vi "诊断标定3 - 副本.vi"(8 "CAN端口":u16(ring), 9 "设备索引号":u16(ring), 10 "CAN卡类型":u32(ring)=21) -> ()   [LabVIEW 2013] (continued)
      w58 = string[][] [["", "", "", "", "", "", "", "", "", "", "", "", "", "", "", "", "", "", "", "", "", "", "", "", "", "", "", "", "", "", "", "", "", "", "", "", "", "", "", "", ""], ["", "", "", "", "", "", "", "", "", "", "", "", "", "", "", "", "", "", "", "", "", "", "", "", "", "", "", "", "", "", "", "", "", "", "", "", "", "", "", "", ""], ["", "", "", "", "", "", "", "", "", "", "", "", "", "", "", "", "", "", "", "", "", "", "", "", "", "", "", "", "", "", "", "", "", "", "", "", "", "", "", "", ""], ["", "", "", "", "", "", "", "", "", "", "", "", "", "", "", "", "", "", "", "", "", "", "", "", "", "", "", "", "", "", "", "", "", "", "", "", "", "", "", "", ""], ["", "", "", "", "", "", "", "", "", "", "", "", "", "", "", "", "", "", "", "", "", "", "", "", "", "", "", "", "", "", "", "", "", "", "", "", "", "", "", "", ""], ["", "", "", "", "", "", "", "", "", "", "", "", "", "", "", "", "", "", "", "", "", "", "", "", "", "", "", "", "", "", "", "", "", "", "", "", "", "", "", "", ""], ["", "", "", "", "", "", "", "", "", "", "", "", "", "", "", "", "", "", "", "", "", "", "", "", "", "", "", "", "", "", "", "", "", "", "", "", "", "", "", "", ""], ["", "", "", "", "", "", "", "", "", "", "", "", "", "", "", "", "", "", "", "", "", "", "", "", "", "", "", "", "", "", "", "", "", "", "", "", "", "", "", "", ""], ["", "", "", "", "", "", "", "", "", "", "", "", "", "", "", "", "", "", "", "", "", "", "", "", "", "", "", "", "", "", "", "", "", "", "", "", "", "", "", "", ""], ["", "", "", "", "", "", "", "", "", "", "", "", "", "", "", "", "", "", "", "", "", "", "", "", "", "", "", "", "", "", "", "", "", "", "", "", "", "", "", "", ""], ["", "", "", "", "", "", "", "", "", "", "", "", "", "", "", "", "", "", "", "", "", "", "", "", "", "", "", "", "", "", "", "", "", "", "", "", "", "", "", "", ""], ["", "", "", "", "", "", "", "", "", "", "", "", "", "", "", "", "", "", "", "", "", "", "", "", "", "", "", "", "", "", "", "", "", "", "", "", "", "", "", "", ""], ["", "", "", "", "", "", "", "", "", "", "", "", "", "", "", "", "", "", "", "", "", "", "", "", "", "", "", "", "", "", "", "", "", "", "", "", "", "", "", "", ""], ["", "", "", "", "", "", "", "", "", "", "", "", "", "", "", "", "", "", "", "", "", "", "", "", "", "", "", "", "", "", "", "", "", "", "", "", "", "", "", "", ""], ["", "", "", "", "", "", "", "", "", "", "", "", "", "", "", "", "", "", "", "", "", "", "", "", "", "", "", "", "", "", "", "", "", "", "", "", "", "", "", "", ""], ["", "", "", "", "", "", "", "", "", "", "", "", "", "", "", "", "", "", "", "", "", "", "", "", "", "", "", "", "", "", "", "", "", "", "", "", "", "", "", "", ""], ["", "", "", "", "", "", "", "", "", "", "", "", "", "", "", "", "", "", "", "", "", "", "", "", "", "", "", "", "", "", "", "", "", "", "", "", "", "", "", "", ""], ["", "", "", "", "", "", "", "", "", "", "", "", "", "", "", "", "", "", "", "", "", "", "", "", "", "", "", "", "", "", "", "", "", "", "", "", "", "", "", "", ""], ["", "", "", "", "", "", "", "", "", "", "", "", "", "", "", "", "", "", "", "", "", "", "", "", "", "", "", "", "", "", "", "", "", "", "", "", "", "", "", "", ""], ["", "", "", "", "", "", "", "", "", "", "", "", "", "", "", "", "", "", "", "", "", "", "", "", "", "", "", "", "", "", "", "", "", "", "", "", "", "", "", "", ""], ["", "", "", "", "", "", "", "", "", "", "", "", "", "", "", "", "", "", "", "", "", "", "", "", "", "", "", "", "", "", "", "", "", "", "", "", "", "", "", "", ""], ["", "", "", "", "", "", "", "", "", "", "", "", "", "", "", "", "", "", "", "", "", "", "", "", "", "", "", "", "", "", "", "", "", "", "", "", "", "", "", "", ""], ["", "", "", "", "", "", "", "", "", "", "", "", "", "", "", "", "", "", "", "", "", "", "", "", "", "", "", "", "", "", "", "", "", "", "", "", "", "", "", "", ""], ["", "", "", "", "", "", "", "", "", "", "", "", "", "", "", "", "", "", "", "", "", "", "", "", "", "", "", "", "", "", "", "", "", "", "", "", "", "", "", "", ""], ["", "", "", "", "", "", "", "", "", "", "", "", "", "", "", "", "", "", "", "", "", "", "", "", "", "", "", "", "", "", "", "", "", "", "", "", "", "", "", "", ""], ["", "", "", "", "", "", "", "", "", "", "", "", "", "", "", "", "", "", "", "", "", "", "", "", "", "", "", "", "", "", "", "", "", "", "", "", "", "", "", "", ""], ["", "", "", "", "", "", "", "", "", "", "", "", "", "", "", "", "", "", "", "", "", "", "", "", "", "", "", "", "", "", "", "", "", "", "", "", "", "", "", "", ""], ["", "", "", "", "", "", "", "", "", "", "", "", "", "", "", "", "", "", "", "", "", "", "", "", "", "", "", "", "", "", "", "", "", "", "", "", "", "", "", "", ""], ["", "", "", "", "", "", "", "", "", "", "", "", "", "", "", "", "", "", "", "", "", "", "", "", "", "", "", "", "", "", "", "", "", "", "", "", "", "", "", "", ""], ["", "", "", "", "", "", "", "", "", "", "", "", "", "", "", "", "", "", "", "", "", "", "", "", "", "", "", "", "", "", "", "", "", "", "", "", "", "", "", "", ""], ["", "", "", "", "", "", "", "", "", "", "", "", "", "", "", "", "", "", "", "", "", "", "", "", "", "", "", "", "", "", "", "", "", "", "", "", "", "", "", "", ""], ["", "", "", "", "", "", "", "", "", "", "", "", "", "", "", "", "", "", "", "", "", "", "", "", "", "", "", "", "", "", "", "", "", "", "", "", "", "", "", "", ""], ["", "", "", "", "", "", "", "", "", "", "", "", "", "", "", "", "", "", "", "", "", "", "", "", "", "", "", "", "", "", "", "", "", "", "", "", "", "", "", "", ""], ["", "", "", "", "", "", "", "", "", "", "", "", "", "", "", "", "", "", "", "", "", "", "", "", "", "", "", "", "", "", "", "", "", "", "", "", "", "", "", "", ""], ["", "", "", "", "", "", "", "", "", "", "", "", "", "", "", "", "", "", "", "", "", "", "", "", "", "", "", "", "", "", "", "", "", "", "", "", "", "", "", "", ""], ["", "", "", "", "", "", "", "", "", "", "", "", "", "", "", "", "", "", "", "", "", "", "", "", "", "", "", "", "", "", "", "", "", "", "", "", "", "", "", "", ""], ["", "", "", "", "", "", "", "", "", "", "", "", "", "", "", "", "", "", "", "", "", "", "", "", "", "", "", "", "", "", "", "", "", "", "", "", "", "", "", "", ""], ["", "", "", "", "", "", "", "", "", "", "", "", "", "", "", "", "", "", "", "", "", "", "", "", "", "", "", "", "", "", "", "", "", "", "", "", "", "", "", "", ""], ["", "", "", "", "", "", "", "", "", "", "", "", "", "", "", "", "", "", "", "", "", "", "", "", "", "", "", "", "", "", "", "", "", "", "", "", "", "", "", "", ""], ["", "", "", "", "", "", "", "", "", "", "", "", "", "", "", "", "", "", "", "", "", "", "", "", "", "", "", "", "", "", "", "", "", "", "", "", "", "", "", "", ""], ["", "", "", "", "", "", "", "", "", "", "", "", "", "", "", "", "", "", "", "", "", "", "", "", "", "", "", "", "", "", "", "", "", "", "", "", "", "", "", "", ""]]
      w47 = TRUE
      w42 = u32 16777215
      w38 = FALSE ("判定2")
      n3 = control-ref of="结果"() -> (w43:refnum<vi>)
      n4 = control-ref of="模块软件版本 2"() -> (w44:refnum<vi>)
      n5 = control-ref of="结果"() -> (w45:refnum<vi>)
      n6 = control-ref of="单选选项2"() -> (w62:refnum<vi>)
      n7 = control-ref of="单选选项1"() -> (w63:refnum<vi>)
      n8 = local write "key names"(string[] []) -> ()
      n9 = property on="项目信息" class="Tbl (严格)"("Disabled"=w39) -> ()  [unwired: 2 in, 2 out]
      n10 = property on="电池实际容量(A)" class="DigNum (严格)"("Disabled"=w39) -> ()  [unwired: 2 in, 2 out]
      n11 = property on="使用者" class="DigNum (严格)"("Disabled"=w39) -> ()  [unwired: 2 in, 2 out]
      n12 = property on="SOH(%)" class="DigNum (严格)"("Disabled"=w39) -> ()  [unwired: 2 in, 2 out]
      n13 = property on="电池额定容量(A)" class="DigNum (严格)"("Disabled"=w39) -> ()  [unwired: 2 in, 2 out]
      n14 = local write "主从选择"(enum32{"主板", "从板"}."主板" ("主从选择")) -> ()
      n15 = property on="SOC(%)" class="DigNum (严格)"("Disabled"=w39) -> ()  [unwired: 2 in, 2 out]
      n16 = local write "等级 2"(T19."从板信息" ("等级 2")) -> ()
      n17 = local write "主板2"(T8."项目信息" ("主从板")) -> ()
      n18 = property class="MCListbox (严格)"(reference=w45, "ItemNames"=w40) -> ()  [unwired: 1 in, 2 out]
      n19 = property class="MCListbox (严格)"(reference=w44, "ItemNames"=w40) -> ()  [unwired: 1 in, 2 out]
      n20 = property class="MCListbox (严格)"(reference=w43, "ItemNames"=w40) -> ()  [unwired: 1 in, 2 out]
      n21 = property class="Bool (严格)"(reference=w62, "BoolText.TextColor"=u32 87470) -> ()  [unwired: 1 in, 2 out]
      n22 = property class="Bool (严格)"(reference=w63, "BoolText.TextColor"=w42) -> ()  [unwired: 1 in, 2 out]
      n23 = property on="从板号" class="DigNum (严格)"("NumText.BGColor"=w42) -> ()  [unwired: 2 in, 2 out]
      n24 = local write "主从板"(enum32{"单选选项2", "单选选项1"}."单选选项1" ("主从板")) -> ()
      n25 = property on="项目信息2" class="Clust (严格)"("DisabledEnum"=w39) -> ()  [unwired: 2 in, 2 out]
      n26 = property on="系统时钟" class="Str"("Disabled"=w39) -> ()  [unwired: 2 in, 2 out]
      n27 = property on="配置文件版本" class="Str"("Disabled"=w39) -> ()  [unwired: 2 in, 2 out]
      n28 = property on="车架(牌)号" class="Str"("Disabled"=w39) -> ()  [unwired: 2 in, 2 out]
      n29 = property on="产品编号" class="Str"("Disabled"=w39) -> ()  [unwired: 2 in, 2 out]
      n30 = local write "判定3"(w47) -> ()
      n31 = local write "清BUFF"(w47) -> ()
      n32 = local write "1"(w47) -> ()
      n33 = property on="从板个数" class="DigNum (严格)"("Visible"=w47) -> ()  [unwired: 2 in, 2 out]
      n34 = property on="从板个数" class="DigNum (严格)"("NumText.BGColor"=u32 16448250) -> ()  [unwired: 2 in, 2 out]
      n35 = Not(x=w47) -> (.not. x?=w66:bool)
      n36 = local write "布尔"(w47) -> ()
      n37 = property on="主板选项" class="Tree (严格)"("Visible"=w47) -> ()  [unwired: 2 in, 2 out]
      n38 = property on="全部写入" class="Bool (严格)"("DisabledEnum"=2) -> ()  [unwired: 2 in, 2 out]
      n39 = property on="从板选项" class="Tree (严格)"("Visible"=w66) -> ()  [unwired: 2 in, 2 out]
      n40 = property on="当前从板板号" class="DigNum (严格)"("Visible"=w66) -> ()  [unwired: 2 in, 2 out]
      n41 = control-ref of="结果"() -> (w53:refnum<vi>)
      n42 = control-ref of="结果"() -> (w50:refnum<vi>)
      n43 = local write "强制停止版本读取"(w38) -> ()
      n44 = local write "强制终止读写标记"(w38) -> ()
      n45 = control-ref of="项目信息"() -> (w51:refnum<vi>)
      n46 = local write "判定2"(w38) -> ()
      n47 = local write "停止"(w38) -> ()
      n48 = local write "控制1"(w38) -> ()
      n49 = local write "消除"(w38) -> ()
      n50 = global write "EV05全局变量1.vi" "授权功能"(w38) -> ()
      n51 = local write "继电器超时处理"(w38) -> ()
      n52 = local write "1 6"(w38) -> ()
      n53 = local write "1 7"(w38) -> ()
      n54 = local write "1 8"(w38) -> ()
      n55 = local write "1 9"(w38) -> ()
      n56 = local write "1 10"(w38) -> ()
      n57 = local write "1 2"(w38) -> ()
      n58 = local write "1 3"(w38) -> ()
      n59 = local write "1 4"(w38) -> ()
      n60 = local write "1 5"(w38) -> ()
      n61 = local write "1 11"(w38) -> ()
      n62 = for {
        N: 150 -> [_]
        tunnel: w53 -> [w92]
        i -> [w90]
        n63 = Bundle(w90, 0) -> (w88:cluster{i32, i32})  [unwired: 1 out]
        n64 = property class="MCListbox (严格)"(reference=w92, "ActiveCell"=w88, "CellBG"=u32 16448250) -> ()  [unwired: 1 in, 2 out]
      }
      n65 = for {
        N: 150 -> [_]
        tunnel: w51 -> [w87]
        i -> [w86]
        n66 = Bundle(w86, 0) -> (w84:cluster{i32, i32})  [unwired: 1 out]
        n67 = property class="Tbl (严格)"(reference=w87, "Active Cell"=w84, "Cell BG Color"=u32 16448250) -> ()  [unwired: 1 in, 2 out]
      }
      n68 = for {
        N: 150 -> [_]
        tunnel: w50 -> [w97]
        i -> [w95]
        n69 = Bundle(w95, 0) -> (w93:cluster{i32, i32})  [unwired: 1 out]
        n70 = property class="MCListbox (严格)"(reference=w97, "ActiveCell"=w93, "CellBG"=u32 16448250) -> ()  [unwired: 1 in, 2 out]
      }
      n71 = stacked-sequence {
        tunnel: [_ w71] -> w46
        frame #0 {
          n72 = local read "设备索引号"() -> (w68:u16)
          n73 = local read "CAN卡类型"() -> (w67:u32)
          n74 = local read "CAN端口"() -> (w69:u16)
          n75 = dll-call lib="PTH1|abs FBluewave New EnergySVN_WorkBMS_Monitor_Bnet01trunkBMS_Monitor_增加二维码data\nkerneldlls\nusbcan.dll" fn="VCI_ClearBuffer"("DeviceType"=w67, "DeviceInd"=w68, "CANInd"=w69) -> (error out=w70:errorcluster)  [unwired: 4 in, 4 out]
          n76 = call <vilib>:"Clear Errors.vi"("error in (no error)"=w70) -> ()  [unwired: 6 in, 1 out]
        }
        frame #1 {
          w78 = u8 0 items=["Normal", "Listen Only"] ("工作方式")
          w77 = u8 1 items=["Dual Filter", "Single Filter"] ("滤波方式")
          n77 = local read "设备索引号"() -> (w73:u16)
          n78 = local read "CAN卡类型"() -> (w72:u32)
          n79 = local read "CAN端口"() -> (w74:u16)
          n80 = call "CAN_Init-8.6.vi"("CAN卡类型"=w72, "设备索引号"=w73, "CAN端口"=w74, "操作类型"=enum16{"初始化CAN", "关闭CAN"}."初始化CAN", "滤波方式"=w77, "Accept Code"=u32 3221225472, "簇"=T21 {"打开CAN"=FALSE, "初始化CAN"=TRUE, "开始CAN"=TRUE, "重启"=FALSE, "关闭CAN"=FALSE}, "Mask Code"=u32 1073741823 ("Accept Code"), "工作方式"=w78, "是否滤波"=TRUE, "滤波选择"=T20 {"fiter_mode"=1, "fiter_endid"=402653184, "fiter_startid"=419430399}) -> ("error out"=w71:errorcluster)  [unwired: 3 in, 5 out]
        }
      }
      n81 = local write "加热继电器(从)"(w38) -> ()
      n82 = local write "风机继电器(从)"(w38) -> ()
      n83 = local write "DO1"(w38) -> ()
      n84 = local write "DO2"(w38) -> ()
      n85 = local write "DO1 2"(w38) -> ()
      n86 = local write "正级继电器"(w38) -> ()
      n87 = local write "负级继电器"(w38) -> ()
      n88 = local write "加热继电器"(w38) -> ()
      n89 = local write "充电继电器"(w38) -> ()
      n90 = local write "风机继电器"(w38) -> ()
      n91 = local write "预充电继电器"(w38) -> ()
      n92 = property on="保存版本信息" class="Bool (严格)"("Visible"=w38) -> ()  [unwired: 2 in, 2 out]
      n93 = property on="单个读取" class="Bool (严格)"("Visible"=w38) -> ()  [unwired: 2 in, 2 out]
      n94 = property on="单个写入" class="Bool (严格)"("Visible"=w38) -> ()  [unwired: 2 in, 2 out]
      n95 = local write "正级继电器 12"(w38) -> ()
      n96 = local write "正级继电器 2"(w38) -> ()
      n97 = local write "正级继电器 3"(w38) -> ()
      n98 = local write "正级继电器 4"(w38) -> ()
      n99 = local write "正级继电器 5"(w38) -> ()
      n100 = local write "正级继电器 6"(w38) -> ()
      n101 = local write "正级继电器 7"(w38) -> ()
      n102 = local write "正级继电器 8"(w38) -> ()
      n103 = local write "正级继电器 9"(w38) -> ()
      n104 = local write "正级继电器 10"(w38) -> ()
      n105 = local write "正级继电器 11"(w38) -> ()
      n106 = property on="从板号" class="DigNum (严格)"("Visible"=w38) -> ()  [unwired: 2 in, 2 out]
      "电池故障" <- w40
      "模块版本值" <- w58
      "硬件版本" <- w59
      "模块版本名称" <- w58
      "平台软件版本" <- w59
      "项目软件版本" <- w59
      "模块个数" <- u8[] [0, 0, 0, 0, 0, 0, 0, 0, 0, 0, 0, 0, 0, 0, 0, 0, 0, 0, 0, 0, 0, 0, 0, 0, 0, 0, 0, 0, 0, 0, 0, 0] ("模块个数")
    }
  }
  n107 = stacked-sequence {
    tunnel: [w98] -> w23
    frame #0 {
      n108 = call <vilib>:"Set Busy.vi"() -> ()  [unwired: 10 in, 2 out]
      n109 = disable-structure shown="禁用" {
        frame Disabled {
          n110 = control-ref of="主板选项"() -> (w217:refnum<vi>)
          n111 = stacked-sequence {
            tunnel: w217 -> [w219 w377 w415]
            frame #0 {
              # "加热和充电控制参数"
              n112 = global read "功能码全局.vi" "主板控制类信息10"() -> (w229:bool[])
              n113 = Index Array(array=w229) -> (element #5=w223:bool, element #6=w221:bool, element #7=w222:bool, element #8=w220:bool)  [unwired: 8 in, 4 out]
              n114 = Not Or(1:w222, 2:w223) -> (0:w228:bool)
              n115 = Not Or(1:w220, 2:w221) -> (0:w226:bool)
              n116 = for {
                N: 8 -> [_]
                tunnel: w219 -> [w349]
                tunnel: w228 -> [w345]
                tunnel: [w344] -> w227
                i -> [w347]
                n117 = Add(x=w347, y=69) -> (x+y=w348:i32)
                n118 = property class="Tree (严格)"(reference=w349, "Active Item Row Number"=w348, "Disabled?"=w345) -> (error out=w344:errorcluster)  [unwired: 1 in, 1 out]
              }
              n119 = for {
                N: 9 -> [_]
                tunnel: w219 -> [w343]
                tunnel: w226 -> [w339]
                tunnel: w227 -> [w338]
                tunnel: [w337] -> w218
                i -> [w341]
                n120 = Add(x=w341, y=77) -> (x+y=w342:i32)
                n121 = property class="Tree (严格)"(reference=w343, error in=w338, "Active Item Row Number"=w342, "Disabled?"=w339) -> (error out=w337:errorcluster)  [unwired: 1 out]
              }
              n122 = stacked-sequence {
                tunnel: w219 -> [w249 _ _]
                tunnel: w218 -> [w248 _ _]
                frame #0 {
                  # "电池信息"
                  n123 = global read "功能码全局.vi" "主板版本号11"() -> (w250:bool[])
                  n124 = global read "功能码全局.vi" "主板项目信息4"() -> (w232:bool[])
                  n125 = Index Array(array=w250) -> (element #1=w246:bool, element #2=w245:bool, element #3=w239:bool, element #4=w233:bool, element #6=w238:bool, element #7=w237:bool, element #8=w236:bool)  [unwired: 8 in, 1 out]
                  n126 = Index Array(array=w232, index=4 ("索引")) -> (element=w230:bool)
                  n127 = Or(x=w239, y=w233) -> (x .or. y?=w234:bool)
                  n128 = Not(x=w237) -> (.not. x?=w241:bool)
                  n129 = Not(x=w236) -> (.not. x?=w240:bool)
                  n130 = Not(x=w238) -> (.not. x?=w242:bool)
                  n131 = property on="硬件版本号" class="Str"("Visible"=w239) -> ()  [unwired: 2 in, 2 out]
                  n132 = property on="读硬件版本号" class="Bool (严格)"("Visible"=w239) -> ()  [unwired: 2 in, 2 out]
                  n133 = property on="项目软件版本号" class="Str"("Visible"=w239) -> ()  [unwired: 2 in, 2 out]
                  n134 = property on="项目软本读取" class="Bool (严格)"("Visible"=w239) -> ()  [unwired: 2 in, 2 out]
                  n135 = property on="继电器屏1 2" class="TabCtl (严格)"("Visible"=w242) -> ()  [unwired: 2 in, 2 out]
                  n136 = property on="均衡屏" class="TabCtl (严格)"("Visible"=w240) -> ()  [unwired: 2 in, 2 out]
                  n137 = property on="继电器屏1 2" class="TabCtl (严格)"("Visible"=w242) -> ()  [unwired: 2 in, 2 out]
                  n138 = property on="DO屏" class="TabCtl (严格)"("Visible"=w241) -> ()  [unwired: 2 in, 2 out]
                  n139 = Compound Arithmetic op=OR(w238, w237, w236) -> (w235:bool)
                  n140 = Not Or(1:w245, 2:w246) -> (0:w244:bool)
                  n141 = stacked-sequence {
                    tunnel: w235 -> [_ w255 _]
                    tunnel: w234 -> [_ _ w259]
                    tunnel: w230 -> [w251 _ _]
                    frame #0 {
                      n142 = case shown="真" w251 {
                        frame False {
                        }
                        frame True {
                          n143 = local write "主界面选项"(enum32{"单选选项1", "单选选项2", "单选选项2 2", "单选选项2 3"}."单选选项2 3" ("主界面选项")) -> ()
                          n144 = local write "面板选择"(T7."高压板校正" ("面板选择")) -> ()
                        }
                      }
                      n145 = control-ref of="单选选项2 3"() -> (w252:refnum<vi>)
                      n146 = property class="Bool (严格)"(reference=w252, "Visible"=w251) -> ()  [unwired: 1 in, 2 out]
                    }
                    frame #1 {
                      n147 = control-ref of="单选选项2 2"() -> (w256:refnum<vi>)
                      n148 = case shown="真" w255 {
                        frame False {
                        }
                        frame True {
                          n149 = local write "主界面选项"(enum32{"单选选项1", "单选选项2", "单选选项2 2", "单选选项2 3"}."单选选项2 2" ("主界面选项")) -> ()
                          n150 = local write "面板选择"(enum32{"读写参数", "版本读取", "其它诊断"}."其它诊断" ("选项卡控件 2")) -> ()
                        }
                      }
                      n151 = property class="Bool (严格)"(reference=w256, "Visible"=w255) -> ()  [unwired: 1 in, 2 out]
                    }
                    frame #2 {
                      n152 = control-ref of="单选选项2"() -> (w260:refnum<vi>)
                      n153 = case shown="真" w259 {
                        frame False {
                        }
                        frame True {
                          n154 = local write "主界面选项"(enum32{"单选选项1", "单选选项2", "单选选项2 2", "单选选项2 3"}."单选选项2" ("主界面选项")) -> ()
                          n155 = local write "面板选择"(enum32{"读写参数", "版本读取", "其它诊断"}."版本读取" ("选项卡控件 2")) -> ()
                        }
                      }
                      n156 = property class="Bool (严格)"(reference=w260, "Visible"=w259) -> ()  [unwired: 1 in, 2 out]
                    }
                  }
                  n157 = for {
                    N: 5 -> [_]
                    tunnel: w249 -> [w269]
                    tunnel: w244 -> [w265]
                    tunnel: w248 -> [w264]
                    tunnel: [w263] -> w247
                    i -> [w267]
                    n158 = Add(x=w267, y=86) -> (x+y=w268:i32)
                    n159 = property class="Tree (严格)"(reference=w269, error in=w264, "Active Item Row Number"=w268, "Disabled?"=w265) -> (error out=w263:errorcluster)  [unwired: 1 out]
                  }
                  n160 = property on="模块软件版本 2" class="MCListbox (严格)"("Visible"=w233) -> ()  [unwired: 2 in, 2 out]
                  n161 = property on="模块软件版本" class="Enum (严格)"("Visible"=w233) -> ()  [unwired: 2 in, 2 out]
                  n162 = property on="平台软件版本号" class="Str"("Visible"=w233) -> ()  [unwired: 2 in, 2 out]
                  n163 = property on="模块版本读取" class="Bool (严格)"("Visible"=w233) -> ()  [unwired: 2 in, 2 out]
                  n164 = property on="平台软件版本读取" class="Bool (严格)"("Visible"=w233) -> ()  [unwired: 2 in, 2 out]
                  n165 = call <vilib>:"Clear Errors.vi"("error in (no error)"=w247) -> ()  [unwired: 6 in, 1 out]
                }
                frame #1 {
                  n166 = global read "功能码全局.vi" "主板项目信息7"() -> (w309:bool[])
                  n167 = global read "功能码全局.vi" "主板控制类信息10"() -> (w305:bool[])
                  n168 = global read "功能码全局.vi" "主板故障阀值9"() -> (w308:bool[])
                  n169 = global read "功能码全局.vi" "主板项目信息4"() -> (w287:bool[])
                  n170 = global read "功能码全局.vi" "主板项目信息5"() -> (w296:bool[])
                  n171 = global read "功能码全局.vi" "主板项目信息6"() -> (w286:bool[])
                  n172 = global read "功能码全局.vi" "主板版本号11"() -> (w295:bool[])
                  n173 = Delete From Array(array=w286, length=1 ("长度"), index=0 ("索引")) -> (deleted portion=w297:bool[], array with subset deleted=w313:bool[])
                  n174 = Index Array(array=w287, index #1=5 ("索引"), index #2=6 ("索引"), index #3=7 ("索引")) -> (element #1=w298:bool, element #2=w314:bool, element #3=w270:bool)
                  n175 = Index Array(array=w295) -> (element #1=w302:bool, element #2=w318:bool)  [unwired: 2 in]
                  n176 = Array Subset(array=w308, index=2 ("索引"), length=3 ("长度")) -> (w300:bool[])
                  n177 = Delete From Array(array=w309, length=3 ("索引"), index=2 ("长度")) -> (deleted portion=w299:bool[], array with subset deleted=w315:bool[])
                  n178 = Array Subset(array=w305, index=4 ("索引"), length=2 ("长度")) -> (w301:bool[])
                  n179 = global read "功能码全局.vi" "18"() -> (w278:bool[])
                  n180 = global read "功能码全局.vi" "16"() -> (w279:bool[])
                  n181 = Insert Into Array(array=w296, new element #1=w297, new element #2=w298, new element #3=w299, new element #4=w300, new element #5=w301, new element #6=w302) -> (w319:bool[])  [unwired: 1 in]
                  n182 = Array Subset(array=w305, index=6 ("索引"), length=2 ("长度")) -> (w317:bool[])
                  n183 = Array Subset(array=w308, index=5 ("索引"), length=3 ("长度")) -> (w316:bool[])
                  n184 = And Array Elements(Boolean array=w319) -> (logical AND=w284:bool)
                  n185 = Array Subset(array=w278, index=0 ("索引"), length=8 ("长度")) -> (w276:bool[])
                  n186 = Array Subset(array=w279, index=4 ("索引"), length=4 ("长度")) -> (w275:bool[])
                  n187 = Or Array Elements(Boolean array=w319) -> (logical OR=w271:bool)
                  n188 = Insert Into Array(array=w313, new element #1=w314, new element #2=w315, new element #3=w316, new element #4=w317, new element #5=w318) -> (w320:bool[])  [unwired: 1 in]
                  n189 = property on="全部读取" class="Bool (严格)"("Visible"=w284) -> ()  [unwired: 2 in, 2 out]
                  n190 = global read "功能码全局.vi" "15"() -> (w277:bool[])
                  n191 = And Array Elements(Boolean array=w320) -> (logical AND=w285:bool)
                  n192 = property on="全部写入" class="Bool (严格)"("Visible"=w285) -> ()  [unwired: 2 in, 2 out]
                  n193 = Or Array Elements(Boolean array=w320) -> (logical OR=w321:bool)
                  n194 = Insert Into Array(array=w277, new element #1=w276, new element #2=w275) -> (w274:bool[])  [unwired: 1 in]
                  n195 = Or Array Elements(Boolean array=w274) -> (logical OR=w273:bool)
                  n196 = Compound Arithmetic op=OR(w270, w271, w321, w273) -> (w322:bool)
                  n197 = case shown="真" w322 {
                    frame False {
                    }
                    frame True {
                      n198 = local write "主界面选项"(enum32{"单选选项1", "单选选项2", "单选选项2 2", "单选选项2 3"}."单选选项1" ("主界面选项")) -> ()
                      n199 = local write "面板选择"(enum32{"读写参数", "版本读取", "其它诊断"}."读写参数" ("选项卡控件 2")) -> ()
                    }
                  }
                  n200 = property on="单选选项1" class="Bool (严格)"("Visible"=w322) -> ()  [unwired: 2 in, 2 out]
                }
                frame #2 {
                  n201 = control-ref of="单选选项2 2"() -> (w329:refnum<vi>)
                  n202 = control-ref of="单选选项2 3"() -> (w325:refnum<vi>)
                  n203 = control-ref of="单选选项2"() -> (w331:refnum<vi>)
                  n204 = control-ref of="单选选项1"() -> (w330:refnum<vi>)
                  n205 = local read "主界面选项"() -> (w334:enum32{"单选选项1", "单选选项2", "单选选项2 2", "单选选项2 3"})
                  n206 = Build Array(w330, w331, w329, w325) -> (w328:refnum<vi>[])
                  n207 = Delete From Array(array=w328, index=w334) -> (deleted portion=w332:refnum<vi>, array with subset deleted=w333:refnum<vi>[])  [unwired: 1 in]
                  n208 = property class="Bool (严格)"(reference=w332, "BoolText.TextColor"=u32 87470) -> ()  [unwired: 1 in, 2 out]
                  n209 = for {
                    tunnel: u32 16777215 -> [w336]
                    tunnel: w333 -> [w335] mode=indexing
                    n210 = property class="Bool (严格)"(reference=w335, "BoolText.TextColor"=w336) -> ()  [unwired: 1 in, 2 out]
                  }
                }
              }
            }
            frame #1 {
              # "项目信息"
              # "SOC"
              # "SOH"
              # "电池额定实际容量"
              # "车牌号"
              # "产品编号"
              # "电压个数"
              # "通道电压数"
              # "温度个数"
              # "电压起始值"
              # "温度起始值"
              # "配置文件版本"
              # "系统时钟"
              # "校正时钟"
              n211 = global read "功能码全局.vi" "主板项目信息5"() -> (w410:bool[])
              n212 = global read "功能码全局.vi" "主板项目信息6"() -> (w409:bool[])
              n213 = global read "功能码全局.vi" "主板项目信息7"() -> (w386:bool[])
              n214 = global read "功能码全局.vi" "主板项目信息4"() -> (w357:bool[])
              n215 = Index Array(array=w410) -> (element #1=w407:bool, element #2=w404:bool, element #3=w401:bool, element #4=w398:bool, element #5=w394:bool, element #6=w392:bool, element #7=w389:bool, element #8=w385:bool)  [unwired: 8 in]
              n216 = Index Array(array=w409) -> (element #1=w382:bool, element #2=w406:bool, element #3=w403:bool, element #4=w400:bool, element #5=w397:bool, element #6=w393:bool, element #7=w391:bool, element #8=w388:bool)  [unwired: 8 in]
              n217 = Index Array(array=w386) -> (element #1=w384:bool, element #2=w381:bool, element #3=w379:bool, element #4=w374:bool, element #5=w371:bool, element #6=w378:bool, element #7=w372:bool, element #8=w370:bool)  [unwired: 8 in]
              n218 = Index Array(array=w357) -> (element #6=w353:bool, element #7=w352:bool, element #8=w356:bool)  [unwired: 8 in, 5 out]
              n219 = Not(x=w356) -> (.not. x?=w355:bool)
              n220 = Not Or(1:w352, 2:w353) -> (0:w351:bool)
              n221 = Not Or(1:w406, 2:w407) -> (0:w369:bool)
              n222 = Not Or(1:w403, 2:w404) -> (0:w368:bool)
              n223 = Not Or(1:w400, 2:w401) -> (0:w367:bool)
              n224 = Not Or(1:w397, 2:w398) -> (0:w366:bool)
              n225 = Not Or(1:w393, 2:w394) -> (0:w365:bool)
              n226 = Not Or(1:w391, 2:w392) -> (0:w364:bool)
              n227 = Not Or(1:w388, 2:w389) -> (0:w363:bool)
              n228 = Not Or(1:w384, 2:w385) -> (0:w362:bool)
              n229 = Not Or(1:w378, 2:w379) -> (0:w360:bool)
              n230 = Not Or(1:w370, 2:w371) -> (0:w358:bool)
              n231 = Not Or(1:w372, 2:w374) -> (0:w359:bool)
              n232 = Not Or(1:w381, 2:w382) -> (0:w361:bool)
              n233 = Compound Arithmetic op=OR(w355, w369, w368, w367, w366, w365, w364, w363, w362, w361, w360, w359, w358) -> (w350:bool)
              "项目信息结果" <- w350
              n234 = property class="Tree (严格)"(reference=w377, "Active Item Row Number"=9 ("活动项:行数"), "Disabled?"=w351, "Active Item Row Number"=1 ("活动项:行数"), "Disabled?"=w350, "Active Item Row Number"=0 ("活动项:行数"), "Disabled?"=w355, "Active Item Row Number"=3 ("活动项:行数"), "Disabled?"=w369, "Active Item Row Number"=4 ("活动项:行数"), "Disabled?"=w368, "Active Item Row Number"=5 ("活动项:行数"), "Disabled?"=w367, "Active Item Row Number"=6 ("活动项:行数"), "Disabled?"=w366, "Active Item Row Number"=7 ("活动项:行数"), "Disabled?"=w365, "Active Item Row Number"=8 ("活动项:行数"), "Disabled?"=w364, "Active Item Row Number"=11 ("活动项:行数"), "Disabled?"=w363, "Active Item Row Number"=12 ("活动项:行数"), "Disabled?"=w362, "Active Item Row Number"=13 ("活动项:行数"), "Disabled?"=w361, "Active Item Row Number"=2 ("活动项:行数"), "Disabled?"=w360, "Active Item Row Number"=10 ("活动项:行数"), "Disabled?"=w359, "Active Item Row Number"=14 ("活动项:行数"), "Disabled?"=w358) -> ()  [unwired: 1 in, 2 out]
            }
            frame #2 {
              w420 = 18
              # "一二三级故障"
              n235 = global read "功能码全局.vi" "主板故障阀值9"() -> (w426:bool[])
              n236 = Index Array(array=w426) -> (element #3=w425:bool, element #4=w422:bool, element #5=w419:bool, element #6=w424:bool, element #7=w421:bool, element #8=w418:bool)  [unwired: 8 in, 2 out]
              n237 = Not Or(1:w424, 2:w425) -> (0:w414:bool)
              n238 = Not Or(1:w421, 2:w422) -> (0:w412:bool)
              n239 = Not Or(1:w418, 2:w419) -> (0:w413:bool)
              n240 = for {
                N: w420 -> [_]
                tunnel: w415 -> [w446]
                tunnel: w414 -> [w442]
                tunnel: [w441] -> w423
                i -> [w444]
                n241 = Add(x=w444, y=15) -> (x+y=w445:i32)
                n242 = property class="Tree (严格)"(reference=w446, "Active Item Row Number"=w445, "Disabled?"=w442) -> (error out=w441:errorcluster)  [unwired: 1 in, 1 out]
              }
              n243 = for {
                N: w420 -> [_]
                tunnel: w415 -> [w440]
                tunnel: w412 -> [w436]
                tunnel: w423 -> [w435]
                tunnel: [w434] -> w417
                i -> [w438]
                n244 = Add(x=w438, y=33) -> (x+y=w439:i32)
                n245 = property class="Tree (严格)"(reference=w440, error in=w435, "Active Item Row Number"=w439, "Disabled?"=w436) -> (error out=w434:errorcluster)  [unwired: 1 out]
              }
              n246 = for {
                N: w420 -> [_]
                tunnel: w415 -> [w433]
                tunnel: w413 -> [w429]
                tunnel: w417 -> [w428]
                tunnel: [w427] -> w416
                i -> [w431]
                n247 = Add(x=w431, y=51) -> (x+y=w432:i32)
                n248 = property class="Tree (严格)"(reference=w433, error in=w428, "Active Item Row Number"=w432, "Disabled?"=w429) -> (error out=w427:errorcluster)  [unwired: 1 out]
              }
              n249 = call <vilib>:"Clear Errors.vi"("error in (no error)"=w416) -> ()  [unwired: 6 in, 1 out]
            }
          }
        }
        frame Enabled {
        }
      }
      n250 = disable-structure shown="禁用" {
        disable-tunnel: [w99 _] -> w98
        frame Disabled {
          n251 = control-ref of="从板选项"() -> (w100:refnum<vi>)
          n252 = stacked-sequence {
            tunnel: w100 -> [w103 w140 w182]
            tunnel: [w101 _ _] -> w99
            frame #0 {
              n253 = global read "功能码全局.vi" "15"() -> (w126:bool[])
              n254 = global read "功能码全局.vi" "16"() -> (w117:bool[])
              n255 = Index Array(array=w126) -> (element #1=w125:bool, element #2=w123:bool, element #3=w121:bool, element #4=w119:bool, element #5=w124:bool, element #6=w122:bool, element #7=w120:bool, element #8=w118:bool)  [unwired: 8 in]
              n256 = Index Array(array=w117) -> (element #5=w108:bool, element #6=w116:bool, element #7=w107:bool, element #8=w115:bool)  [unwired: 8 in, 4 out]
              n257 = Not Or(1:w115, 2:w116) -> (0:w105:bool)
              n258 = Not Or(1:w107, 2:w108) -> (0:w106:bool)
              n259 = Not Or(1:w124, 2:w125) -> (0:w111:bool)
              n260 = Not Or(1:w122, 2:w123) -> (0:w112:bool)
              n261 = Not Or(1:w120, 2:w121) -> (0:w113:bool)
              n262 = Not Or(1:w118, 2:w119) -> (0:w114:bool)
              n263 = Compound Arithmetic op=OR(w111, w112, w113, w114, w105) -> (w110:bool)
              "从板项目信息" <- w110
              n264 = property class="Tree (严格)"(reference=w103, "Active Item Row Number"=1 ("活动项:行数"), "Disabled?"=w110, "Active Item Row Number"=2 ("活动项:行数"), "Disabled?"=w111, "Active Item Row Number"=3 ("活动项:行数"), "Disabled?"=w112, "Active Item Row Number"=4 ("活动项:行数"), "Disabled?"=w113, "Active Item Row Number"=5 ("活动项:行数"), "Disabled?"=w114, "Active Item Row Number"=0 ("活动项:行数"), "Disabled?"=w106) -> (error out=w102:errorcluster)  [unwired: 1 in, 1 out]
              n265 = for {
                N: 8 -> [_]
                tunnel: w103 -> [w138]
                tunnel: w105 -> [w134]
                tunnel: w102 -> [w133]
                tunnel: [w132] -> w101
                i -> [w136]
                n266 = Add(x=w136, y=6) -> (x+y=w137:i32)
                n267 = property class="Tree (严格)"(reference=w138, error in=w133, "Active Item Row Number"=w137, "Disabled?"=w134) -> (error out=w132:errorcluster)  [unwired: 1 out]
              }
              n268 = call <vilib>:"Clear Errors.vi"("error in (no error)"=w101) -> ()  [unwired: 6 in, 1 out]
            }
            frame #1 {
              w151 = 8
              n269 = global read "功能码全局.vi" "18"() -> (w160:bool[])
              n270 = Index Array(array=w160) -> (element #1=w143:bool, element #2=w144:bool, element #3=w159:bool, element #4=w154:bool, element #5=w148:bool, element #6=w158:bool, element #7=w153:bool, element #8=w147:bool)  [unwired: 8 in]
              n271 = Not Or(1:w144, 2:w143) -> (0:w139:bool)
              n272 = property class="Tree (严格)"(reference=w140, "Active Item Row Number"=46 ("活动项:行数"), "Disabled?"=w139, "Active Item Row Number"=47 ("活动项:行数"), "Disabled?"=w139, "Active Item Row Number"=48 ("活动项:行数"), "Disabled?"=w139) -> ()  [unwired: 1 in, 2 out]
              n273 = Not Or(1:w147, 2:w148) -> (0:w146:bool)
              n274 = Not Or(1:w158, 2:w159) -> (0:w157:bool)
              n275 = Not Or(1:w153, 2:w154) -> (0:w152:bool)
              n276 = for {
                N: w151 -> [_]
                tunnel: w140 -> [w181]
                tunnel: w157 -> [w177]
                tunnel: "error out" -> [w176]
                tunnel: [w175] -> w155
                i -> [w179]
                n277 = Add(x=w179, y=14) -> (x+y=w180:i32)
                n278 = property class="Tree (严格)"(reference=w181, error in=w176, "Active Item Row Number"=w180, "Disabled?"=w177) -> (error out=w175:errorcluster)  [unwired: 1 out]
              }
              n279 = for {
                N: w151 -> [_]
                tunnel: w140 -> [w174]
                tunnel: w152 -> [w170]
                tunnel: w155 -> [w169]
                tunnel: [w168] -> w150
                i -> [w172]
                n280 = Add(x=w172, y=22) -> (x+y=w173:i32)
                n281 = property class="Tree (严格)"(reference=w174, error in=w169, "Active Item Row Number"=w173, "Disabled?"=w170) -> (error out=w168:errorcluster)  [unwired: 1 out]
              }
              n282 = for {
                N: w151 -> [_]
                tunnel: w140 -> [w167]
                tunnel: w146 -> [w163]
                tunnel: w150 -> [w162]
                tunnel: [w161] -> w149
                i -> [w165]
                n283 = Add(x=w165, y=30) -> (x+y=w166:i32)
                n284 = property class="Tree (严格)"(reference=w167, error in=w162, "Active Item Row Number"=w166, "Disabled?"=w163) -> (error out=w161:errorcluster)  [unwired: 1 out]
              }
              n285 = call <vilib>:"Clear Errors.vi"("error in (no error)"=w149) -> ()  [unwired: 6 in, 1 out]
            }
            frame #2 {
              n286 = global read "功能码全局.vi" "23"() -> (w206:bool[])
              n287 = global read "功能码全局.vi" "24"() -> (w204:bool[])
              n288 = Index Array(array=w206) -> (element #3=w205:bool, element #4=w202:bool, element #5=w200:bool, element #6=w198:bool, element #7=w196:bool, element #8=w194:bool)  [unwired: 8 in, 2 out]
              n289 = Index Array(array=w204) -> (element #3=w203:bool, element #4=w201:bool, element #5=w199:bool, element #6=w197:bool, element #7=w195:bool, element #8=w193:bool)  [unwired: 8 in, 2 out]
              n290 = Not Or(1:w203, 2:w205) -> (0:w192:bool)
              n291 = Not Or(1:w201, 2:w202) -> (0:w187:bool)
              n292 = Not Or(1:w199, 2:w200) -> (0:w188:bool)
              n293 = Not Or(1:w197, 2:w198) -> (0:w189:bool)
              n294 = Not Or(1:w195, 2:w196) -> (0:w191:bool)
              n295 = Not Or(1:w193, 2:w194) -> (0:w190:bool)
              n296 = Build Array(w192, w192, w191, w190, w189, w188, w187) -> (w185:bool[])
              n297 = And Array Elements(Boolean array=w185) -> (logical AND=w186:bool)
              n298 = Insert Into Array(array=w185, index=0 ("索引"), new element=w186) -> (w183:bool[])
              n299 = for {
                N: 8 -> [_]
                tunnel: w182 -> [w216]
                tunnel: w183 -> [w212] mode=indexing
                tunnel: errorcluster {"status"=FALSE, "code"=0, "source"=""} ("error out 2") -> [w211]
                tunnel: [w210] -> w208
                i -> [w214]
                n300 = Add(x=w214, y=38) -> (x+y=w215:i32)
                n301 = property class="Tree (严格)"(reference=w216, error in=w211, "Active Item Row Number"=w215, "Disabled?"=w212) -> (error out=w210:errorcluster)  [unwired: 1 out]
              }
              n302 = call <vilib>:"Clear Errors.vi"("error in (no error)"=w208) -> ()  [unwired: 6 in, 1 out]
            }
          }
        }
        frame Enabled {
        }
      }
    }
  }
  n303 = local write "项目信息 2"(string[][] [["电压个数", "36"], ["温度个数", "45"], ["第一个保险通道", "0"], ["第一个保险位置", "0"], ["第二个保险通道", "0"], ["第二个保险位置", "0"], ["第三个保险通道", "0"], ["第三个保险位置", "0"], ["第四个保险通道", "0"], ["第四个保险位置", "0"], ["第五个保险通道", "0"], ["第五个保险位置", "0"], ["第六个保险通道", "0"], ["第六个保险位置", "0"], ["第七个保险通道", "0"], ["第七个保险位置", "0"], ["第八个保险通道", "0"], ["第八个保险位置", "0"], ["第九个保险通道", "0"], ["第九个保险位置", "0"], ["第十个保险通道", "0"], ["第十个保险位置", "0"], ["第1通道电压个数", "11"], ["第2通道电压个数", "12"], ["第3通道电压个数", "12"], ["第4通道电压个数", "12"], ["第5通道电压个数", "12"]] ("项目信息 2")) -> ()
  n304 = Index Array(array=w13, index (col)=0 ("索引 (行)")) -> (element=w16:string[])  [unwired: 1 in]
  n305 = Index Array(array=w13, index (col)=1 ("禁用的索引 (列)")) -> (element=w6:string[])  [unwired: 1 in]
  n306 = local read "从板个数"() -> (w8:dbl)
  n307 = Array Subset(array=w16, index=0 ("索引"), length=w8) -> (w15:string[])
  n308 = Array Subset(array=w16, index=10 ("索引"), length=w8) -> (w14:string[])
  n309 = Array Subset(array=w6, index=0 ("索引"), length=w8) -> (w12:string[])
  n310 = Array Subset(array=w6, index=10 ("索引"), length=w8) -> (w7:string[])
  n311 = Insert Into Array(array=w15, new element=w14) -> (w5:string[])  [unwired: 1 in]
  n312 = Insert Into Array(array=w12, new element=w7) -> (w4:string[])  [unwired: 1 in]
  n313 = stacked-sequence {
    tunnel: w20 -> [_]
    tunnel: w23 -> [_]
    frame #0 {
      n314 = call <vilib>:"Unset Busy.vi"() -> ()  [unwired: 11 in, 1 out]
    }
  }
  n315 = Build Array(w5, w4) -> (w3:string[][])
  n316 = local write "停止"(FALSE ("停止")) -> ()
  n317 = Transpose 2D Array(2D array=w3) -> (transposed array=w2:string[][])
  n318 = Obtain Queue(name (unnamed)=w37, element data type=w37, error in (no error)=w20) -> (queue out=w36:refnum<queue>, error out=w35:errorcluster)  [unwired: 2 in, 1 out]
  n319 = local write "项目信息"(w2) -> ()
  n320 = Obtain Queue(element data type="读参数") -> (queue out=w25:refnum<queue>, error out=w24:errorcluster)  [unwired: 4 in, 1 out]
  n321 = while {
    tunnel: w25 -> [w458]
    tunnel: w24 -> [w457]
    tunnel: [w456] -> w28
    tunnel: [w455] -> w27
    tunnel: w20 -> [_]
    tunnel: w23 -> [w447]
    stop <- w454 stop-if-true
    n322 = local read "停止"() -> (w454:bool)
    n323 = local read "设备索引号"() -> (w451:u16)
    n324 = local read "CAN卡类型"() -> (w452:u32)
    n325 = local read "CAN端口"() -> (w450:u16)
    n326 = call "receiver-8.6.vi"("错误输入（无错误）"=w447, "CAN端口"=w450, "设备索引号"=w451, "CAN卡类型"=w452) -> ("错误输出"=w453:errorcluster, "输出簇"=w449:T22, "接收成功"=w448:bool)  [unwired: 3 out]
    n327 = call <vilib>:"Clear Errors.vi"("error in (no error)"=w453) -> ()  [unwired: 6 in, 1 out]
    n328 = case shown="真" w448 {
      tunnel: w457 -> [w459 w465]
      tunnel: w449 -> [_ w464]
      tunnel: w458 -> [w460 w463]
      tunnel: [w460 w462] -> w456
      tunnel: [w459 w461] -> w455
      frame False {
      }
      frame True {
        n329 = Enqueue Element(queue=w463, element=w464, error in (no error)=w465) -> (queue out=w462:refnum<queue>, error out=w461:errorcluster)  [unwired: 2 out]
      }
    }
  }
  n330 = while {
    tunnel: w25 -> [w473]
    tunnel: w24 -> [w472]
    stop <- w466 stop-if-true
    n331 = local read "停止"() -> (w466:bool)
    n332 = local read "控制1"() -> (w468:bool)
    n333 = Dequeue Element(queue=w473, timeout in ms (-1)=200 ("超时毫秒(-1)"), error in (no error)=w472) -> (element=w471:T3, error out=w470:errorcluster)  [unwired: 2 out]
    n334 = case shown="无错误" w470 {
      tunnel: w471 -> [w478 _]
      tunnel: "写?" -> [w475 _]
      tunnel: w468 -> [w474 _]
      frame No Error {
        n335 = Unbundle(w478) -> ("return type"=w477:u32, "pReceive"=w476:T23)
        n336 = for {
          N: w477 -> [_]
          tunnel: w476 -> [w482] mode=indexing
          tunnel: w475 -> [w480]
          tunnel: w474 -> [w479]
          n337 = Unbundle By Name(w482) -> ("ID"=w483:u32)
          n338 = call "ID解析.vi"("ID"=w483) -> ("PDU(1)"=w481:i32)  [unwired: 10 out]
          n339 = case shown="18" w481 {
            tunnel: w482 -> [_ w493]
            tunnel: w480 -> [_ w485]
            tunnel: w479 -> [_ w484]
            frame 0, Default {
            }
            frame 24 {
              n340 = local read "主从选择"() -> (w486:enum32{"主板", "从板"})
              n341 = local read "设备索引号"() -> (w489:u16)
              n342 = local read "CAN卡类型"() -> (w488:u32)
              n343 = local read "CAN端口"() -> (w490:u16)
              n344 = disable-structure shown="禁用" {
                disable-tunnel: w493 -> [w496 _]
                frame Disabled {
                  n345 = call "标定授权读取.vi"("VCI_Receive"=w496) -> ()  [unwired: 1 out]
                }
                frame Enabled {
                }
              }
              n346 = case shown="\"从板\"" w486 {
                tunnel: [0 ("FUNC") w495] -> w487
                frame "主板", Default {
                }
                frame "从板" {
                  n347 = local read "从板号"() -> (w495:u8)
                }
              }
              n348 = local read "面板选择"() -> (w492:T7)
              n349 = case shown="\"读写参数\", 默认" w492 {
                tunnel: w485 -> [w501 _ _ _]
                tunnel: "命令" -> [w502 w605 w860 w1000]
                tunnel: w486 -> [w511 _ w868 w1008]
                tunnel: w493 -> [_ _ _ _]
                tunnel: w493 -> [w507 w606 w862 w1002]
                tunnel: w490 -> [w506 w607 w863 w1003]
                tunnel: w489 -> [w505 w608 w864 w1004]
                tunnel: w488 -> [w504 w609 w865 w1005]
                tunnel: w487 -> [w503 _ w861 w1001]
                tunnel: w484 -> [w497 _ _ _]
                frame "读写参数", Default {
                  n350 = local read "命令序号"() -> (w500:u8)
                  n351 = call "多帧接收机制(EV05).vi"("can卡类型"=w504, "设备索引号"=w505, "CAN端口"=w506, "VCI_Receive"=w507, "命令"=w502, "板号"=w503, "写?"=w501, "命令序号"=w500) -> ("错误信号"=w498:bool, "错误代码"=w510:i32, "输出数组"=w509:u8[], "读错误代码"=w499:u8[], "结束信号"=w508:bool)  [unwired: 7 out]
                  n352 = case shown="假" w501 {
                    tunnel: w508 -> [w521 w588]
                    tunnel: w510 -> [w520 w587]
                    tunnel: w500 -> [w519 _]
                    tunnel: w509 -> [w518 _]
                    tunnel: w502 -> [w517 _]
                    tunnel: w511 -> [w515 w586]
                    tunnel: w499 -> [w514 _]
                    tunnel: w498 -> [w513 _]
                    tunnel: w497 -> [w512 _]
                    frame False {
                      # "读参数"
                      n353 = And(x=w512, y=w521) -> (x .and. y?=w516:bool)
                      n354 = case shown="真" w516 {
                        tunnel: w520 -> [_ w532]
                        tunnel: w519 -> [_ w531]
                        tunnel: w518 -> [_ w530]
                        tunnel: w517 -> [_ w529]
                        tunnel: w515 -> [_ w525]
                        tunnel: w514 -> [_ w523]
                        tunnel: w513 -> [_ w524]
                        frame False {
                        }
                        frame True {
                          n355 = case shown="假" w524 {
                            tunnel: w532 -> [w543 _]
                            tunnel: w531 -> [w542 _]
                            tunnel: w530 -> [w541 _]
                            tunnel: w529 -> [w539 _]
                            tunnel: w525 -> [w535 _]
                            tunnel: w523 -> [_ w571]
                            frame False {
                              n356 = case shown="\"主板\", 默认" w535 {
                                tunnel: [w545 _] -> w538
                                tunnel: [_ w559] -> w537
                                tunnel: [w544 _] -> w534
                                frame "主板", Default {
                                n357 = stacked-sequence {
                                tunnel: [_ w558] -> w545
                                tunnel: [w546 _] -> w544
                                frame #0 {
                                n358 = control-ref of="一级故障"() -> (w552:refnum<vi>)
                                n359 = control-ref of="一级故障 2"() -> (w554:refnum<vi>)
                                n360 = control-ref of="一级故障 3"() -> (w555:refnum<vi>)
                                n361 = control-ref of="加热控制参数"() -> (w556:refnum<vi>)
                                n362 = control-ref of="充电控制参数"() -> (w557:refnum<vi>)
                                n363 = control-ref of="电池信息"() -> (w550:refnum<vi>)
                                n364 = control-ref of="项目信息"() -> (w553:refnum<vi>)
                                n365 = control-ref of="项目信息2"() -> (w551:refnum<vi>)
                                n366 = control-ref of="高压参数"() -> (w549:refnum<vi>)
                                n367 = local read "主板数据"() -> (w548:T4)
                                n368 = Bundle(cluster=w548, "项目信息"=w553, "一级故障 4"=w551, "一级故障"=w552, "一级故障 2"=w554, "一级故障 3"=w555, "加热控制参数"=w556, "充电控制参数"=w557, "高压参数"=w549, "电池信息"=w550) -> (w547:T4)
                                n369 = control-ref of="二维码信息"() -> (w546:refnum<vi>)
                                n370 = local write "主板数据"(w547) -> ()
                                }
                                frame #1 {
                                n371 = control-ref of="主板数据"() -> (w558:refnum<vi>)
                                }
                                }
                                }
                                frame "从板" {
                                n372 = stacked-sequence {
                                tunnel: [_ w570] -> w559
                                frame #0 {
                                n373 = control-ref of="从板号"() -> (w564:refnum<vi>)
                                n374 = control-ref of="项目信息 2"() -> (w565:refnum<vi>)
                                n375 = control-ref of="电池组信息"() -> (w563:refnum<vi>)
                                n376 = control-ref of="加热控制参数"() -> (w566:refnum<vi>)
                                n377 = control-ref of="一级故障(从板)"() -> (w567:refnum<vi>)
                                n378 = control-ref of="二级故障(从板)"() -> (w568:refnum<vi>)
                                n379 = control-ref of="三级故障(从板)"() -> (w569:refnum<vi>)
                                n380 = control-ref of="均衡参数"() -> (w562:refnum<vi>)
                                n381 = local read "从板信息"() -> (w561:T2)
                                n382 = Bundle(cluster=w561, "从板号"=w564, "项目信息 2"=w565, "加热控制参数"=w566, "一级故障(从板)"=w567, "二级故障(从板)"=w568, "三级故障(从板)"=w569, "电池组信息(从板)"=w563, "均衡参数"=w562) -> (w560:T2)
                                n383 = local write "从板信息"(w560) -> ()
                                }
                                frame #1 {
                                n384 = control-ref of="从板信息"() -> (w570:refnum<vi>)
                                }
                                }
                                }
                              }
                              n385 = control-ref of="二维码信息 2"() -> (w533:refnum<vi>)
                              n386 = control-ref of="结果"() -> (w540:refnum<vi>)
                              n387 = control-ref of="从板个数"() -> (w536:refnum<vi>)
                              n388 = call "输出数据解析.vi"("主板引用"=w538, "从板引用"=w537, "板选择"=w535, "二维码信息"=w534, "错误代码"=w543, "命令序号"=w542, "输入数组"=w541, "命令"=w539, "进度引用"=w540, "从板个数"=w536, "从板二维码信息"=w533) -> ()  [unwired: 5 out]
                            }
                            frame True {
                              n389 = Index Array(array=w571, index #1=0 ("索引"), index #2=1 ("索引")) -> (element #1=w574:u8, element #2=w575:u8)
                              n390 = Join Numbers(hi=w574, lo=w575) -> ((hi.lo)=w573:u16)
                              n391 = Number To Hexadecimal String(2:w573) -> (0:w572:string)  [unwired: 1 out]
                              n392 = control-ref of="结果"() -> (w580:refnum<vi>)
                              n393 = Concatenate Strings("0x" ("字符串"), w572) -> (w581:string)
                              n394 = Build Array(w581) -> (w582:string[])
                              n395 = call "表格编辑.vi"("新元素/子数组"=w582, "活动单元格:单元格背景色"=u32 16740749, "MCListbox引用句柄"=w580) -> ()  [unwired: 9 out]
                            }
                          }
                          n396 = global write "EV05全局变量1.vi" "流控帧 2"(FALSE ("流控帧 2")) -> ()
                          n397 = global write "EV05全局变量1.vi" "输出数组"(i32[] []) -> ()
                          n398 = local write "控制1"(FALSE ("控制1")) -> ()
                          n399 = local write "消除"(FALSE ("消除")) -> ()
                        }
                      }
                    }
                    frame True {
                      # "写参数判定"
                      n400 = And(x="控制1", y=w588) -> (x .and. y?=w585:bool)
                      n401 = case shown="真" w585 {
                        tunnel: w587 -> [_ w595]
                        tunnel: w586 -> [_ w592]
                        frame False {
                        }
                        frame True {
                          n402 = call <vilib>:"Unset Busy.vi"() -> ()  [unwired: 2 in, 10 out]
                          n403 = case shown="\"主板\", 默认" w592 {
                            tunnel: [w596 w597] -> w594
                            frame "主板", Default {
                              n404 = local read "主板选项"() -> (w596:string)
                            }
                            frame "从板" {
                              n405 = local read "从板选项"() -> (w597:string)
                            }
                          }
                          n406 = control-ref of="结果"() -> (w593:refnum<vi>)
                          n407 = call "输入数据判定.vi"("主从选择"=w592, "主板选项"=w594, "进度引用"=w593, "错误代码"=w595) -> ()  [unwired: 2 in, 6 out]
                          n408 = global write "EV05全局变量1.vi" "流控帧 2"(FALSE ("流控帧 2")) -> ()
                          n409 = local write "控制1"(FALSE ("控制1")) -> ()
                          n410 = local write "消除"(FALSE ("消除")) -> ()
                        }
                      }
                      n411 = global write "EV05全局变量1.vi" "输出数组"(i32[] []) -> ()
                    }
                  }
                }
                frame "版本读取" {
                  n412 = local read "命令序号"() -> (w598:u8)
                  n413 = local read "从板板号"() -> (w601:u8)
                  n414 = local read "控制1"() -> (w602:bool)
                  n415 = call "多帧接收机制(EV05).vi"("can卡类型"=w609, "设备索引号"=w608, "CAN端口"=w607, "VCI_Receive"=w606, "命令"=w605, "板号"=w601, "命令序号"=w598) -> ("错误信号"=w599:bool, "输出数组"=w610:u8[], "读错误代码"=w600:u8[], "结束信号"=w604:bool)  [unwired: 1 in, 8 out]
                  n416 = And(x=w602, y=w604) -> (x .and. y?=w603:bool)
                  n417 = case shown="真" w603 {
                    tunnel: w610 -> [_ w618]
                    tunnel: w598 -> [_ w617]
                    tunnel: w605 -> [_ w616]
                    tunnel: w600 -> [_ w612]
                    tunnel: w599 -> [_ w611]
                    frame False {
